vi "Quick stop pdo.vi"(8 "error in (no error)":errorcluster) -> (0 "error out":errorcluster)   [LabVIEW 2014]
uses:
  <vilib>/CANopenLib/CANOPEN.llb/CANopen Convert To Data [U16].vi
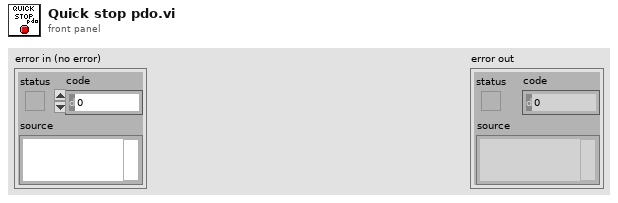
[diagram p1: front panel]
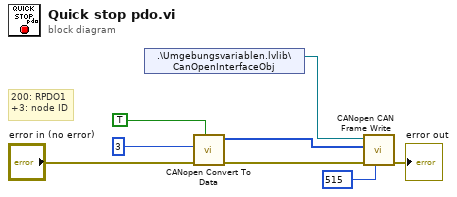
[diagram p0: block diagram]
diagram:
  # "200: RPDO1\n+3: node ID"
  n1 = shared-variable ".\\Umgebungsvariablen.lvlib\\CanOpenInterfaceObj"() -> (w8:refnum<k20>)  [unwired: 1 in, 1 out]
  n2 = call-poly <vilib>:"CANopen Convert To Data.vi"("trim"=TRUE, "error in (no error)"="error in (no error)", "unsigned 16-bit integer"=u16 3) -> ("error out"=w3:errorcluster, "CANopen data out"=w6:u8[])  [unwired: 7 in]
  n3 = call <vilib>:"CANopen CAN Frame Write.vi"("COB-ID (0)"=u32 515, "error in (no error)"=w3, "CAN message data"=w6, "interface object  in"=w8) -> ("error out"=→"error out":errorcluster)  [unwired: 6 in, 1 out]
